vi "Advance past whitespace.vi"(4 "Past Colon":bool, 6 "Past Comma":bool, 7 "JSON":string, 9 "Offset":i32, 11 "Parser State in":T1=enum."Leading Whitespace") -> (0 "Comma Not Found":bool, 1 "Offset of first non-whitespace":i32, 3 "Parser State":T1)   [LabVIEW 2019, in "JSONtext.lvlib"]
uses:
  JSONtext.lvlib
  Parsing State.ctl
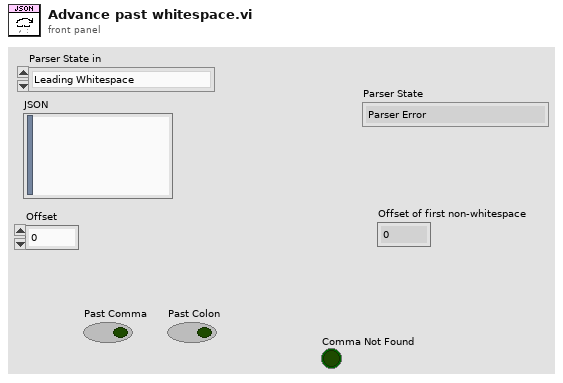
[diagram p1: front panel]
types:
  T1 = typedef "JSONtext.lvlib/Parsing State.ctl" = enum16{"Parser Error", "Object", "Array", "String", "Number/Other", "Leading Whitespace", "Object end", "Array end", "Value end"}
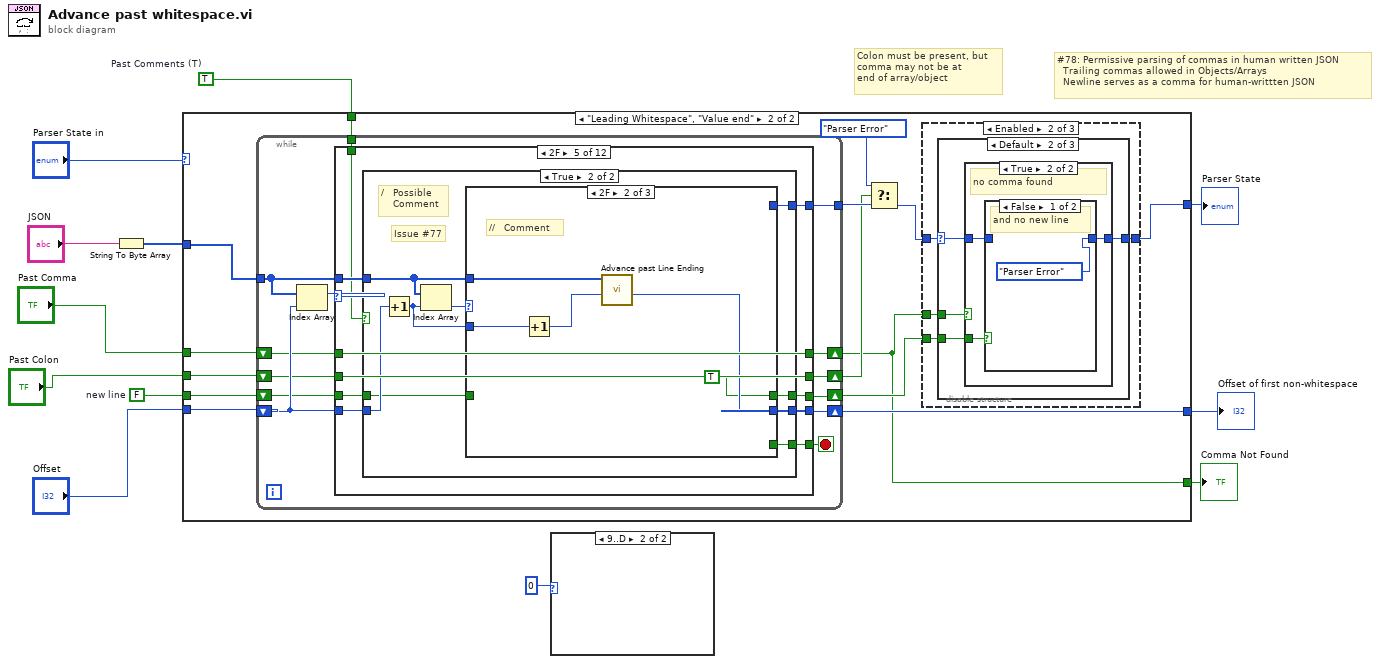
[diagram p0: block diagram]
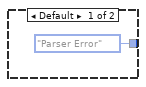
[diagram p6: hidden frame]
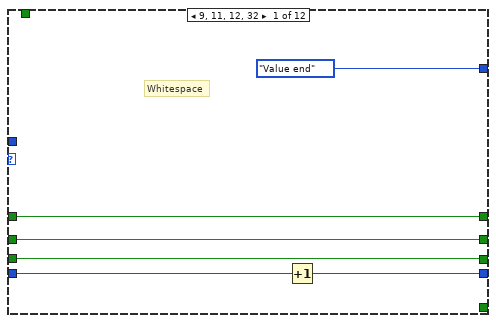
[diagram p12: hidden frame]
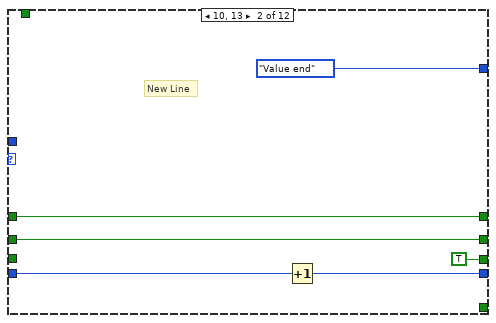
[diagram p13: hidden frame]
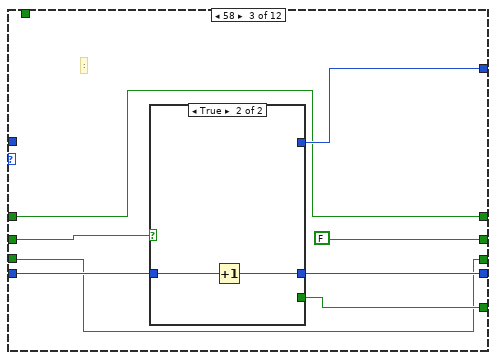
[diagram p14: hidden frame]
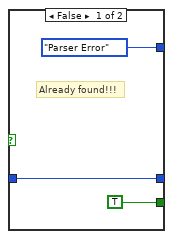
[diagram p15: hidden frame]
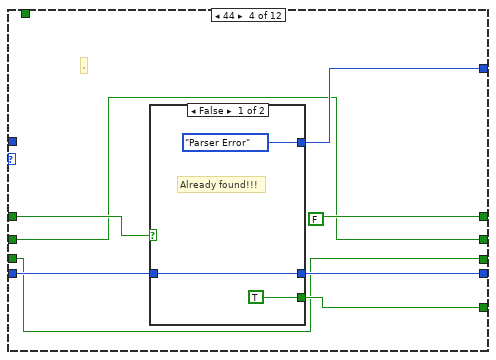
[diagram p16: hidden frame]
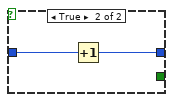
[diagram p17: hidden frame]
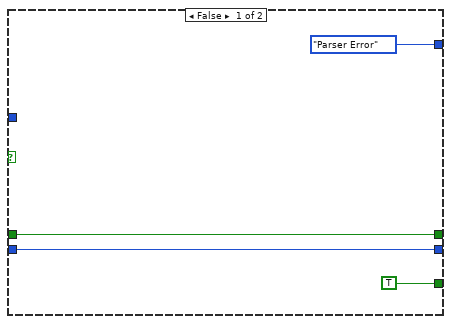
[diagram p18: hidden frame]
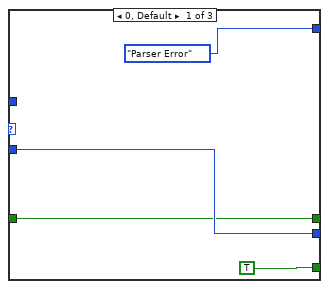
[diagram p19: hidden frame]
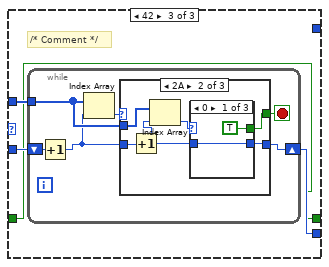
[diagram p20: hidden frame]
diagram:
  w3 = FALSE  # new line
  w4 = TRUE  # Past Comments (T)
  # "#78: Permissive parsing of commas in human written JSON\n  Trailing commas allowed in Objects/Arrays\n  Newline serves as a comma for human-writtten JSON"
  # "Colon must be present, but\ncomma may not be at\nend of array/object"
  n1 = String To Byte Array(string="JSON") -> (unsigned byte array=w6:u8[])
  n2 = case shown="\"Leading Whitespace\", \"Value end\"" "Parser State in" {
    selector: "Parser State in" -> [w14 _]
    tunnel: [w14 w28] -> w12
    tunnel: [w13 w27] -> w11
    tunnel: "Offset" -> [w13 w26]
    tunnel: w6 -> [_ w19]
    tunnel: "Past Comma" -> [_ w25]
    tunnel: "Past Colon" -> [_ w24]
    tunnel: w4 -> [_ w18]
    tunnel: w3 -> [_ w17]
    tunnel: [_ w15] -> w1
    frame "Parser Error", Default {
    }
    frame "Leading Whitespace", "Value end" {
      n3 = while {
        tunnel: w19 -> [w56]
        shift-right: [w61] -> w27
        shift-left: w26 -> [w62]
        tunnel: [w64] -> w23
        shift-right: [w60] -> w15
        shift-left: w25 -> [w59]
        shift-right: [w57] -> w21
        shift-left: w24 -> [w58]
        tunnel: w18 -> [w55]
        shift-right: [w53] -> w16
        shift-left: w17 -> [w54]
        stop <- w63 stop-if-true
        n4 = Index Array(array=w56, index=w62) -> (element=w65:u8)
        n5 = case shown="2F" w65 {
          tunnel: [Parsing_State."Value end" Parsing_State."Value end" w83 w96 w108 Parsing_State."String" Parsing_State."Number/Other" Parsing_State."Array" Parsing_State."Array end" Parsing_State."Object" Parsing_State."Object end" Parsing_State."Parser Error"] -> w64
          tunnel: [_ _ w82 w95 w107 TRUE TRUE TRUE TRUE TRUE TRUE TRUE] -> w63
          tunnel: w62 -> [w71 w77 w85 w98 w111 w165 w171 w177 w183 w189 w195 w203]
          tunnel: [w70 w76 w84 w97 w109 w165 w171 w177 w183 w189 w195 w203] -> w61
          tunnel: [w68 w74 w79 FALSE ("Allow Comma") w113 w164 w170 w176 w182 w188 w194 w200] -> w60
          tunnel: w59 -> [w68 w74 w79 w94 w113 w164 w170 w176 w182 w188 w194 w200]
          tunnel: [w67 w73 FALSE ("Allow Comma") w92 w112 w163 w169 w175 w181 w187 w193 w199] -> w57
          tunnel: w58 -> [w67 w73 w81 w92 w112 w163 w169 w175 w181 w187 w193 w199]
          tunnel: w56 -> [_ _ _ _ w110 _ _ _ _ _ _ _]
          tunnel: w55 -> [_ _ _ _ w106 _ _ _ _ _ _ _]
          tunnel: w54 -> [w66 _ w78 w91 w105 w162 w168 w174 w180 w186 w192 w198]
          tunnel: [w66 TRUE w78 w91 w104 w162 w168 w174 w180 w186 w192 w198] -> w53
          frame 9, 11, 12, 32 {
            # "Whitespace"
            n6 = Increment(x=w71) -> (x+1=w70:i32)
          }
          frame 10, 13 {
            # "New Line"
            n7 = Increment(x=w77) -> (x+1=w76:i32)
          }
          frame 58 {
            # ":"
            n8 = case shown="True" w81 {
              tunnel: w85 -> [w87 w90]
              tunnel: [w87 w89] -> w84
              tunnel: [Parsing_State."Parser Error" _] -> w83
              tunnel: [TRUE _] -> w82
              frame False {
                # "Already found!!!"
              }
              frame True {
                n9 = Increment(x=w90) -> (x+1=w89:i32)
              }
            }
          }
          frame 44 {
            # ","
            n10 = case shown="False" w94 {
              tunnel: w98 -> [w100 w103]
              tunnel: [w100 w102] -> w97
              tunnel: [Parsing_State."Parser Error" _] -> w96
              tunnel: [TRUE _] -> w95
              frame False {
                # "Already found!!!"
              }
              frame True {
                n11 = Increment(x=w103) -> (x+1=w102:i32)
              }
            }
          }
          frame 47 {
            n12 = case shown="True" w106 {
              tunnel: w111 -> [w116 w126]
              tunnel: w110 -> [_ w124]
              tunnel: [w116 w122] -> w109
              tunnel: [Parsing_State."Parser Error" ("t") w121] -> w108
              tunnel: [TRUE w120] -> w107
              tunnel: w105 -> [w114 w119]
              tunnel: [w114 w118] -> w104
              frame False {
              }
              frame True {
                # "Issue #77"
                # "/   Possible \n    Comment"
                n13 = Increment(x=w126) -> (x+1=w123:i32)
                n14 = Index Array(array=w124, index=w123) -> (element=w125:u8)
                n15 = case shown="2F" w125 {
                  tunnel: w124 -> [_ w135 w139]
                  tunnel: w123 -> [w128 w134 w137]
                  tunnel: [w128 w133 w138] -> w122
                  tunnel: [Parsing_State."Parser Error" ("t") _ _] -> w121
                  tunnel: [TRUE _ _] -> w120
                  tunnel: w119 -> [w127 _ w136]
                  tunnel: [w127 TRUE w136] -> w118
                  frame 0, Default {
                  }
                  frame 47 {
                    # "//   Comment"
                    n16 = Increment(x=w134) -> (x+1=w132:i32)
                    n17 = call "Advance past Line Ending.vi"("Offset"=w132, "JSON"=w135) -> ("Offset after Line Ending"=w133:i32)  [unwired: 9 in]
                  }
                  frame 42 {
                    # "/* Comment */"
                    n18 = while {
                      tunnel: w139 -> [w142]
                      shift-right: [w143] -> w138
                      shift-left: w137 -> [w141]
                      stop <- w144 stop-if-true
                      n19 = Increment(x=w141) -> (x+1=w140:i32)
                      n20 = Index Array(array=w142, index=w140) -> (element=w145:u8)
                      n21 = case shown="2A" w145 {
                        tunnel: w140 -> [w146 w150 w161]
                        tunnel: [_ w147 TRUE] -> w144
                        tunnel: [w146 w148 w161] -> w143
                        tunnel: w142 -> [_ w149 _]
                        frame Default {
                        }
                        frame 42 {
                          n22 = Increment(x=w150) -> (x+1=w151:i32)
                          n23 = Index Array(array=w149, index=w151) -> (element=w152:u8)
                          n24 = case shown="0" w152 {
                            tunnel: [TRUE FALSE TRUE] -> w147
                            tunnel: w151 -> [w154 w156 w158]
                            tunnel: [w154 w156 w157] -> w148
                            frame 0 {
                            }
                            frame Default {
                            }
                            frame 47 {
                              n25 = Increment(x=w158) -> (x+1=w157:i32)
                            }
                          }
                        }
                        frame 0 {
                        }
                      }
                    }
                  }
                }
              }
            }
          }
          frame 34 {
          }
          frame 43, 45, 46, 48..57, 69, 73, 78, 101, 102, 110, 116 {
          }
          frame 91 {
          }
          frame 93 {
          }
          frame 123 {
          }
          frame 125 {
          }
          frame Default {
          }
        }
      }
      n26 = Select(t=Parsing_State."Parser Error", s=w21, f=w23) -> (s? t:f=w20:T1)
      n27 = disable-structure shown="Enabled" {
        disable-tunnel: [w31 w40 _] -> w28
        disable-tunnel: w15 -> [w30 w39 _]
        disable-tunnel: w20 -> [w29 w38 _]
        disable-tunnel: w16 -> [_ w37 _]
        frame Disabled {
          n28 = case shown="True" w30 {
            tunnel: w29 -> [w32 w34]
            tunnel: [w32 w33] -> w31
            frame False {
            }
            frame True {
              # "Comma not found is OK\nonly if Object or Array end"
              n29 = case shown="\"Object end\", \"Array end\"" w34 {
                selector: w34 -> [_ w36]
                tunnel: [Parsing_State."Parser Error" w36] -> w33
                frame Default {
                }
                frame "Object end", "Array end" {
                }
              }
            }
          }
        }
        frame Enabled {
          n30 = case shown="Default" w38 {
            selector: w38 -> [w41 w43 w52]
            tunnel: [w41 w44 w52] -> w40
            tunnel: w39 -> [_ w45 _]
            tunnel: w37 -> [_ w42 _]
            frame "Parser Error" {
            }
            frame Default {
              n31 = case shown="True" w45 {
                tunnel: [w46 w47] -> w44
                tunnel: w43 -> [w46 w48]
                tunnel: w42 -> [_ w49]
                frame False {
                }
                frame True {
                  # "no comma found"
                  n32 = case shown="False" w49 {
                    tunnel: w48 -> [_ w51]
                    tunnel: [Parsing_State."Parser Error" ("t") w51] -> w47
                    frame False {
                      # "and no new line"
                    }
                    frame True {
                      # "Counts as a\ncomma"
                      # "but new line"
                    }
                  }
                }
              }
            }
            frame "Object end", "Array end" {
              # "At Object or Array end\nwe usually have no comma\nbut accept a comma"
            }
          }
        }
        frame Disabled {
        }
      }
    }
  }
  "Parser State" <- w12
  "Offset of first non-whitespace" <- w11
  "Comma Not Found" <- w1
  n33 = case shown="9..D" 0 {
    frame 0, Default {
    }
    frame 9..13 {
    }
  }
